vi "Set Greeting Ref.vi"(8 "error in (no error)":errorcluster, 10 "Last Greeting":refnum<vi>, 11 "WebSocket Test UI Refs in":refnum<class "WebSocket Test UI Refs.lvclass">) -> (0 "error out":errorcluster, 3 "WebSocket Test UI Refs out":refnum<class "WebSocket Test UI Refs.lvclass">)   [LabVIEW 2020, in "WebSocket Test UI Refs.lvclass"]
uses:
  WebSocket Test UI Refs.lvclass
  WebSocket Test UI Refs.lvclass/WebSocket Test UI Refs.ctl
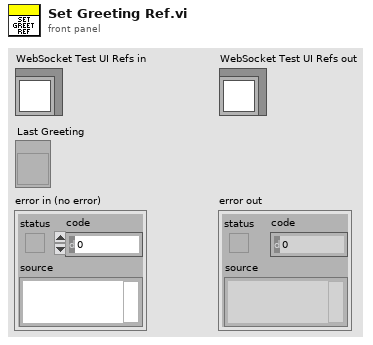
[diagram p1: front panel]
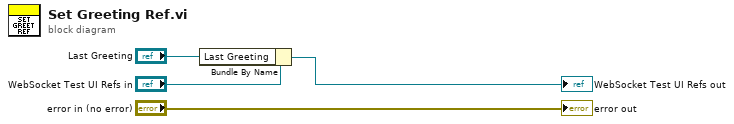
[diagram p0: block diagram]
diagram:
  n1 = Bundle By Name(cluster="WebSocket Test UI Refs in", "Last Greeting"="Last Greeting") -> (→"WebSocket Test UI Refs out":refnum<class "WebSocket Test UI Refs.lvclass">)
  "error out" <- "error in (no error)"
